vi "Scratchpad.vi"() -> ()   [LabVIEW 2020]
uses:
  FlexBlock Node/FlexBlock.xnode
  <extravilib>/ChannelInstances/Flex-dbl/))Channel.ctl
  <extravilib>/ChannelInstances/Flex-dbl.lvlib
  <extravilib>/ChannelInstances/Flex-c(dbl,dbl,a[.](dbl))/))Channel.ctl
  <extravilib>/ChannelInstances/Flex-c(dbl,dbl,a[.](dbl)).lvlib
  <extravilib>/ChannelInstances/Flex-t'Function Generator.lvlib-Shape.ctl'.lvlib
  FlexBlocks/Shape.ctl
  Workers/Function Generator/Function Generator.lvlib
panel:
  in  "Phase":dbl
  in  "Offset":dbl
  in  "stop":bool
  in  "Shape":T1
  in  "Amplitude":dbl(slide) scale=0.0..10.0
  in  "Frequency":dbl(slide) scale=1.0..100.0
  out "Graph":cluster{"t0":dbl, "dt":dbl, "y":dbl[]}(graph)
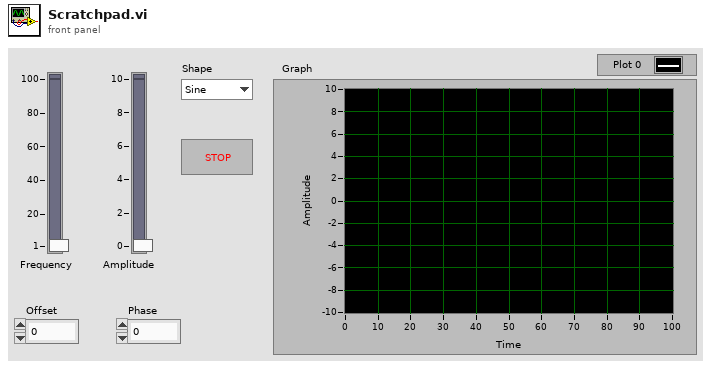
[diagram p1: front panel]
types:
  T1 = typedef "Function Generator.lvlib/Shape.ctl" = enum16{"Sine", "Square", "Triangle", "Saw"}
  T2 = typedef "Flex-dbl.lvlib/))Channel.ctl" = refnum<queue>
  T3 = typedef "Flex-t'Function Generator.lvlib-Shape.ctl'.lvlib/))Channel.ctl" = refnum<queue>
  T4 = typedef "Flex-c(dbl,dbl,a[.](dbl)).lvlib/))Channel.ctl" = refnum<queue>
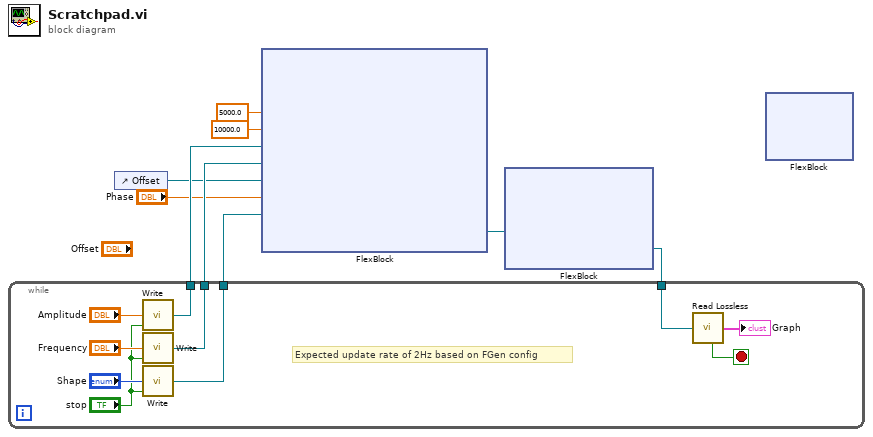
[diagram p0: block diagram]
diagram:
  n1 = control-ref of="Offset"() -> (w4:refnum<vi>)
  n2 = xnode "FlexBlock"() -> ()
  n3 = while {
    tunnel: [w19] -> w7
    tunnel: [w16] -> w6
    tunnel: [w14] -> w5
    tunnel: w1 -> [w11]
    stop <- w10 stop-if-true
    # "Expected update rate of 2Hz based on FGen config"
    n4 = call <extravilib>:"Write.vi"("element"="Amplitude", "Close? (F)"="stop") -> ("channel"=w16:T2)  [unwired: 3 in, 2 out]
    n5 = call <extravilib>:"Write.vi"("element"="Frequency", "Close? (F)"="stop") -> ("channel"=w19:T2)  [unwired: 3 in, 2 out]
    n6 = call <extravilib>:"Write.vi"("element"="Shape", "Close? (F)"="stop") -> ("channel"=w14:T3)  [unwired: 3 in, 2 out]
    n7 = call <extravilib>:"Read Lossless.vi"("FlexChannel"=w11) -> ("Element"=→"Graph":cluster{"t0":dbl, "dt":dbl, "y":dbl[]}, "Closed?"=w10:bool)  [unwired: 6 in, 1 out]
  }
  n8 = xnode "FlexBlock"("Sample Count"=5000.0, "Sample Frequency"=10000.0, "Amplitude"=w6, "Frequency"=w7, "Offset"=w4, "Phase"="Phase", "Shape"=w5) -> ("Out"=w2:T4)
  n9 = xnode "FlexBlock"("In"=w2) -> ("Out"=w1:T4)
